vi "Get Default Name and Path.vi"(8 "error in (no error)":errorcluster) -> (0 "error out":errorcluster, 2 "Project root folder":path, 3 "Project name":string)   [LabVIEW 2013, in "Project Wizard.lvlib"]
uses:
  Project Wizard.lvlib
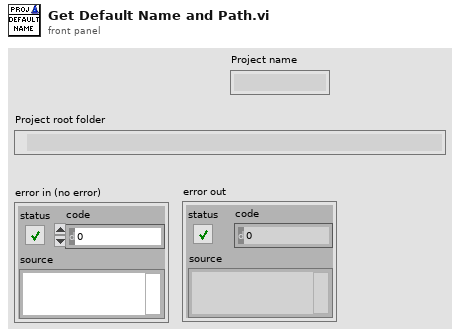
[diagram p1: front panel]
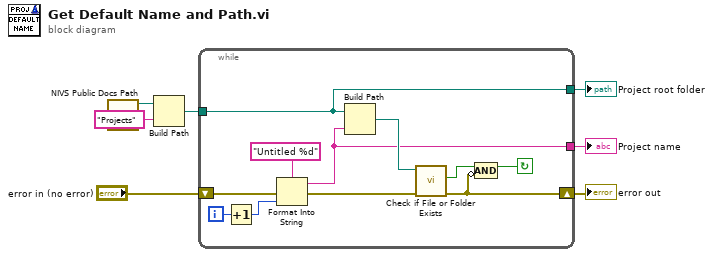
[diagram p0: block diagram]
diagram:
  n1 = call "NIVS Public Docs Path.vi"() -> ("NI VeriStand publid docs path"=w7:path)  [unwired: 11 in]
  n2 = Build Path(base path=w7, name or relative path="Projects") -> (appended path=w4:path)
  n3 = while {
    shift-right: [w8] -> w1
    shift-left: "error in (no error)" -> [w18]
    tunnel: w4 -> [w11]
    tunnel: [w12] -> w3
    tunnel: [w11] -> w2
    i -> [w17]
    stop <- w9 continue-if-true
    n4 = Increment(x=w17) -> (x+1=w16:i32)
    n5 = Format Into String(format string="Untitled %d", error in=w18, w16) -> (resulting string=w12:string, error out=w14:errorcluster)  [unwired: 1 in]
    n6 = Build Path(base path=w11, name or relative path=w12) -> (appended path=w13:path)
    n7 = call <vilib>:"Check if File or Folder Exists.vi"("error in (no error)"=w14, "path"=w13) -> ("error out"=w8:errorcluster, "file or folder exists?"=w10:bool)  [unwired: 7 in, 1 out]
    n8 = Compound Arithmetic op=AND(w10, invert w8) -> (w9:bool)
  }
  "error out" <- w1
  "Project name" <- w3
  "Project root folder" <- w2
